vi "MoveAbsolute.vi"(8 "Error In":errorcluster, 10 "Move Abs Value":dbl, 11 "Thorlabs In":refnum<class "Thorlabs.lvclass">) -> (0 "Error Out":errorcluster, 3 "Thorlabs Out":refnum<class "Thorlabs.lvclass">)   [LabVIEW 2018, in "Thorlabs.lvlib" / "Thorlabs.lvclass"]
doc: "This VI moves the Axis to the absolute location.\n\nCreator: Slade Jeppesen\nCreated Date: 09/29/20"
uses:
  Thorlabs.lvclass
  Thorlabs.lvclass/Thorlabs.ctl
  C:/AME Test Engineering/LabVIEW/PPLs/Axis/DLLs/ThorLabs.MotionControl.KCube.DCServoCLI.dll
  PPLs/Axis/DLLs/ThorLabs.MotionControl.KCube.DCServoCLI.dll
  d5833a60-5d64-4e7a-b253-a555de51ce61.vi
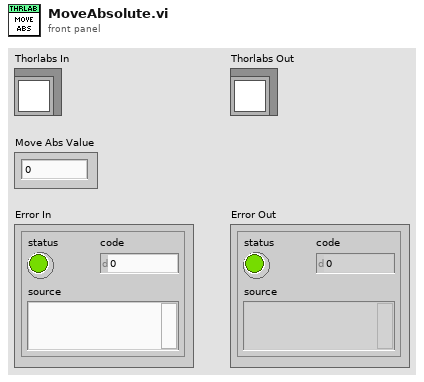
[diagram p1: front panel]
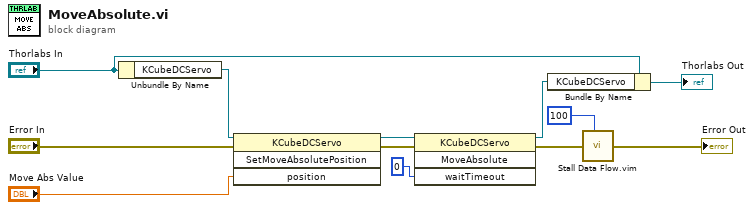
[diagram p0: block diagram]
diagram:
  n1 = Unbundle By Name("Thorlabs In") -> ("KCubeDCServo"=w12:refnum<k24>)
  n2 = invoke class="KCubeDCServo" method="SetMoveAbsolutePosition"(reference=w12, error in="Error In", "position"="Move Abs Value") -> (reference out=w10:refnum<k24>, error out=w11:errorcluster)  [unwired: 1 in, 2 out]
  n3 = invoke class="KCubeDCServo" method="MoveAbsolute"(reference=w10, error in=w11, "waitTimeout"=0) -> (reference out=w7:refnum<k24>, error out=w3:errorcluster)  [unwired: 1 in, 2 out]
  n4 = Bundle By Name(cluster="Thorlabs In", "KCubeDCServo"=w7) -> (→"Thorlabs Out":refnum<class "Thorlabs.lvclass">)
  n5 = call "Stall Data Flow.vim"("value in"=w3, "milliseconds to wait"=u32 100) -> ("value out"=→"Error Out":errorcluster)  [unwired: 1 out]
